vi "MongoDB.DocumentInsert.vi"(8 "error in (no error)":errorcluster, 10 "JSON Document":string, 11 "MongoDB.Collection in":refnum<class "MongoDB.Collection.lvclass">) -> (0 "error out":errorcluster, 2 "output cluster":T1, 3 "MongoDB.Collection out":refnum<class "MongoDB.Collection.lvclass">)   [LabVIEW 2014, in "MongoDB.Collection.lvclass"]
uses:
  MongoDB.Collection.lvclass
  C:/Users/Richard/Documents/GitHub/mongo-labview-driver/CSharp/bin/MongoDB.Bson.dll
  CSharp/bin/MongoDB.Bson.dll
  MongoDB.Collection.lvclass/MongoDB.Collection.ctl
  C:/Users/Richard/Documents/GitHub/mongo-labview-driver/CSharp/bin/MongoDB.Driver.Legacy.dll
  CSharp/bin/MongoDB.Driver.Legacy.dll
  C:/Users/Richard/Documents/GitHub/mongo-labview-driver/CSharp/bin/MongoDB.Driver.Core.dll
  CSharp/bin/MongoDB.Driver.Core.dll
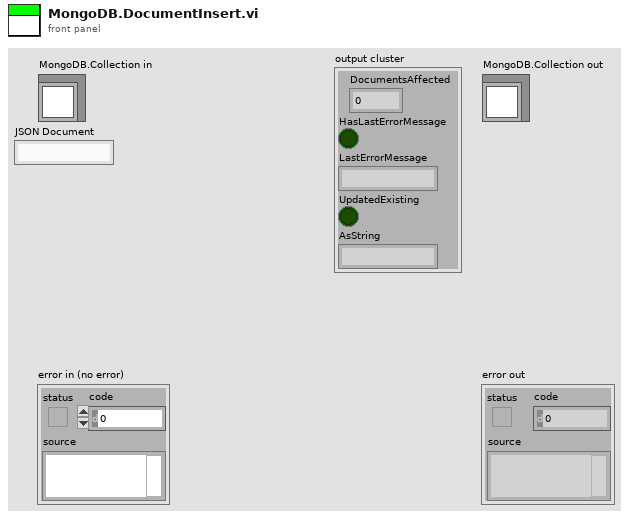
[diagram p1: front panel]
types:
  T1 = cluster{"DocumentsAffected":i64, "HasLastErrorMessage":bool, "LastErrorMessage":string, "UpdatedExisting":bool, "AsString":string}
  T2 = cluster{"DocumentsAffected":i64, "HasLastErrorMessage":bool, "LastErrorMessage":string, "UpdatedExisting":bool, "ToString":string}
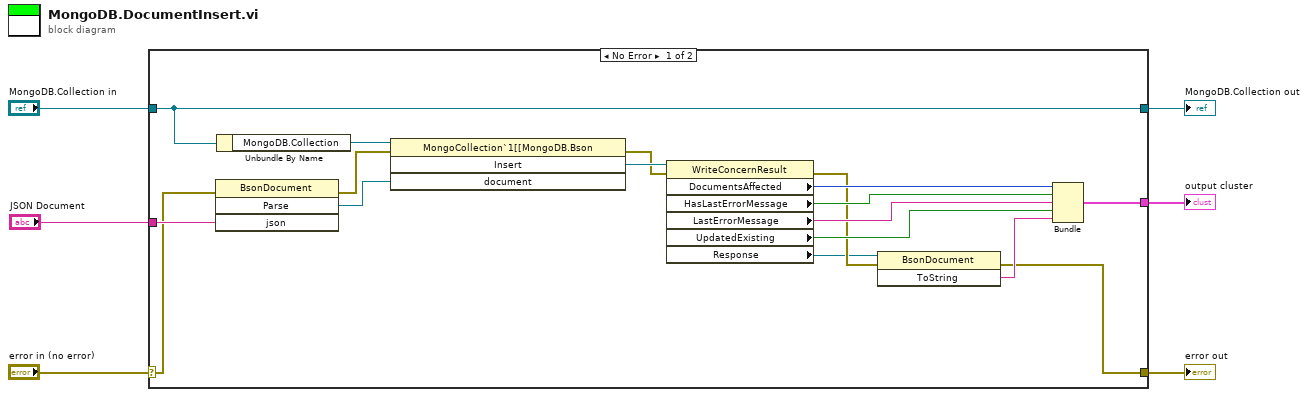
[diagram p0: block diagram]
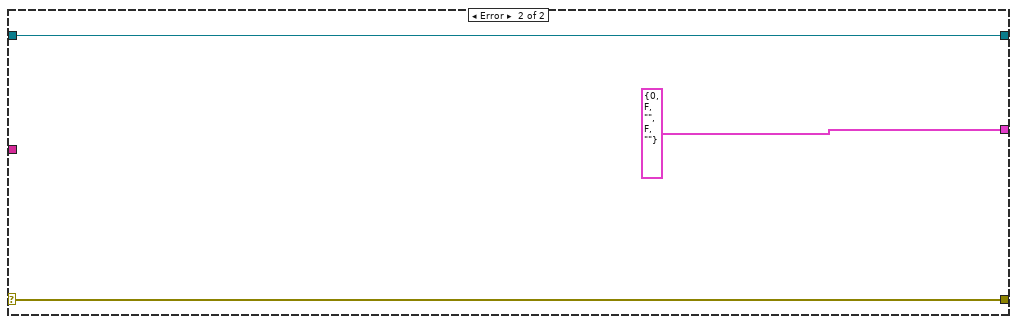
[diagram p2: hidden frame]
diagram:
  n1 = case shown="No Error" "error in (no error)" {
    selector: "error in (no error)" -> [w19 w26]
    tunnel: [w7 w26] -> w5
    tunnel: [w23 w25] -> w3
    tunnel: "MongoDB.Collection in" -> [w23 w25]
    tunnel: "JSON Document" -> [w20 _]
    tunnel: [w8 T1 {"DocumentsAffected"=0, "HasLastErrorMessage"=FALSE, "LastErrorMessage"="", "UpdatedExisting"=FALSE, "AsString"=""}] -> w1
    frame No Error {
      n2 = invoke class="BsonDocument" method="Parse"(error in=w19, "json"=w20) -> (error out=w18:errorcluster, "Parse"=w21:refnum<k24>)  [unwired: 2 in, 2 out]
      n3 = Unbundle By Name(w23) -> ("MongoDB.Collection"=w22:refnum<k24>)
      n4 = invoke class="MongoCollection`1[[MongoDB.Bson" method="Insert"(reference=w22, error in=w18, "document"=w21) -> (error out=w16:errorcluster, "Insert"=w17:refnum<k24>)  [unwired: 1 in, 2 out]
      n5 = property class="WriteConcernResult"(reference=w17, error in=w16) -> (error out=w11:errorcluster, "DocumentsAffected"=w15:i64, "HasLastErrorMessage"=w14:bool, "LastErrorMessage"=w13:string, "UpdatedExisting"=w12:bool, "Response"=w10:refnum<k24>)  [unwired: 1 out]
      n6 = invoke class="BsonDocument" method="ToString"(reference=w10, error in=w11) -> (error out=w7:errorcluster, "ToString"=w9:string)  [unwired: 1 in, 1 out]
      n7 = Bundle("DocumentsAffected"=w15, "HasLastErrorMessage"=w14, "LastErrorMessage"=w13, "UpdatedExisting"=w12, "ToString"=w9) -> (w8:T2)  [unwired: 1 in]
    }
    frame Error {
    }
  }
  "error out" <- w5
  "MongoDB.Collection out" <- w3
  "output cluster" <- w1
